vi "CT_OrganizeDischargeData.vi"(1 "Cap Discharge Array In":T1=[{"cap number and switch SN array"=[{"Switch SN"="SN_U", "Cap Number"=109.0}], "Rog"=enum."F240", "Delay"=enum."PreForm", "Power Supply"=enum."PS1"}, {"cap number and switch SN array"=[{"Switch SN"="SN_U", "Cap Number"=110.0}], "Rog"=enum."F180", "Delay"=enum."DB16", "Power Supply"=enum."PS2"}, {"cap number and switch SN array"=[{"Switch SN"="SN_U", "Cap Number"=111.0}], "Rog"=enum."F300", "Delay"=enum."DB16", "Power Supply"=enum."PS2"}, {"cap number and switch SN array"=[{"Switch SN"="SN_U", "Cap Number"=112.0}], "Rog"=enum."F000", "Delay"=enum."DB16", "Power Supply"=enum."PS2"}, {"cap number and switch SN array"=[{"Switch SN"="SN_U", "Cap Number"=113.0}], "Rog"=enum."F060", "Delay"=enum."DB16", "Power Supply"=enum."PS2"}, {"cap number and switch SN array"=[{"Switch SN"="SN_U", "Cap Number"=114.0}], "Rog"=enum."F120", "Delay"=enum."DB16", "Power Supply"=enum."PS2"}, {"cap number and switch SN array"=[{"Switch SN"="SN_U", "Cap Number"=115.0}], "Rog"=enum."F120", "Delay"=enum."DB16", "Power Supply"=enum."PS2"}, {"cap number and switch SN array"=[{"Switch SN"="SN_U", "Cap Number"=116.0}], "Rog"=enum."F060", "Delay"=enum."DB16", "Power Supply"=enum."PS2"}, {"cap number and switch SN array"=[{"Switch SN"="SN_U", "Cap Number"=117.0}], "Rog"=enum."F000", "Delay"=enum."DB16", "Power Supply"=enum."PS2"}, {"cap number and switch SN array"=[{"Switch SN"="SN_U", "Cap Number"=118.0}], "Rog"=enum."F300", "Delay"=enum."DB16", "Power Supply"=enum."PS2"}, {"cap number and switch SN array"=[{"Switch SN"="SN_U", "Cap Number"=119.0}], "Rog"=enum."F180", "Delay"=enum."DB16", "Power Supply"=enum."PS2"}, {"cap number and switch SN array"=[{"Switch SN"="SN_U", "Cap Number"=120.0}], "Rog"=enum."F240", "Delay"=enum."DB16", "Power Supply"=enum."PS2"}, {"cap number and switch SN array"=[{"Switch SN"="SN_U", "Cap Number"=121.0}], "Rog"=enum."F240", "Delay"=enum."DB16", "Power Supply"=enum."PS3"}, {"cap number and switch SN array"=[{"Switch SN"="SN_U", "Cap Number"=122.0}], "Rog"=enum."F300", "Delay"=enum."DB16", "Power Supply"=enum."PS3"}, {"cap number and switch SN array"=[{"Switch SN"="SN_U", "Cap Number"=123.0}], "Rog"=enum."F180", "Delay"=enum."DB16", "Power Supply"=enum."PS3"}, {"cap number and switch SN array"=[{"Switch SN"="SN_U", "Cap Number"=124.0}], "Rog"=enum."F240", "Delay"=enum."DB16", "Power Supply"=enum."PS3"}, {"cap number and switch SN array"=[{"Switch SN"="SN_U", "Cap Number"=125.0}], "Rog"=enum."DISC", "Delay"=enum."DB16", "Power Supply"=enum."PS3"}, {"cap number and switch SN array"=[{"Switch SN"="SN_U", "Cap Number"=126.0}], "Rog"=enum."F000", "Delay"=enum."DB16", "Power Supply"=enum."PS3"}, {"cap number and switch SN array"=[{"Switch SN"="SN_U", "Cap Number"=127.0}], "Rog"=enum."F060", "Delay"=enum."DB16", "Power Supply"=enum."PS3"}, {"cap number and switch SN array"=[{"Switch SN"="SN_U", "Cap Number"=128.0}], "Rog"=enum."DISC", "Delay"=enum."DB16", "Power Supply"=enum."PS3"}]) -> (0 "Discharge File Data":string[][](array[string]))   [LabVIEW 2016]
uses:
  CapDischargeCluster.ctl
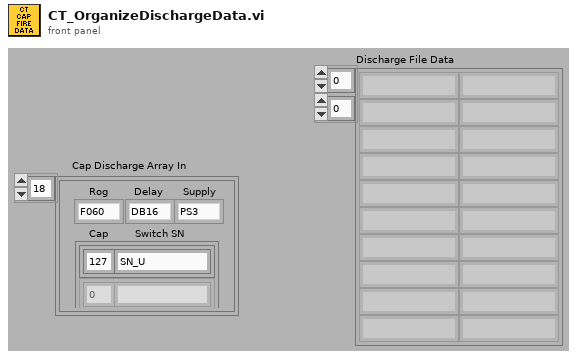
[diagram p1: front panel]
types:
  T1 = typedef "CapDischargeCluster.ctl" = cluster{"cap number and switch SN array":cluster{"Switch SN":string, "Cap Number":dbl}[], "Rog":enum16{"F000", "F060", "F120", "F180", "F240", "F300", "A015", "A045", "A075", "A105", "A135", "A165", "A195", "A225", "A255", "A285", "A315", "A345", "Snip", "DISC"}, "Delay":enum16{"DB00", "DB01", "DB02", "DB03", "DB04", "DB05", "DB06", "DB07", "DB08", "DB09", "DB10", "DB11", "DB12", "DB13", "DB14", "DB15", "DB16", "DB17", "DB18", "DB19", "DB20", "DB21", "DB22", "DB23", "DB24", "DB25", "DB26", "DB27", "DB28", "DB29", "DB30", "PreForm", "Form"}, "Power Supply":enum16{"PS1", "PS2", "PS3", "PS5", "PS6", "PS4"}}[]
  T2 = enum16{"F000", "F060", "F120", "F180", "F240", "F300", "A015", "A045", "A075", "A105", "A135", "A165", "A195", "A225", "A255", "A285", "A315", "A345", "Snip", "DISC"}
  T3 = enum16{"DB00", "DB01", "DB02", "DB03", "DB04", "DB05", "DB06", "DB07", "DB08", "DB09", "DB10", "DB11", "DB12", "DB13", "DB14", "DB15", "DB16", "DB17", "DB18", "DB19", "DB20", "DB21", "DB22", "DB23", "DB24", "DB25", "DB26", "DB27", "DB28", "DB29", "DB30", "PreForm", "Form"}
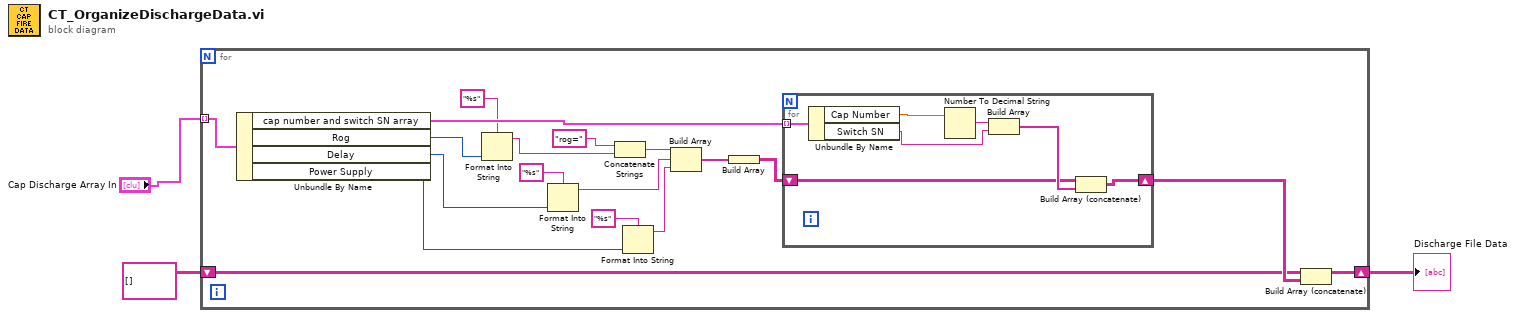
[diagram p0: block diagram]
diagram:
  n1 = for {
    tunnel: "Cap Discharge Array In" -> [w21] mode=indexing
    shift-right: [w18] -> w2
    shift-left: string[][] [] -> [w17]
    n2 = Unbundle By Name(w21) -> ("cap number and switch SN array"=w20:cluster{"Switch SN":string, "Cap Number":dbl}[], "Rog"=w16:T2, "Delay"=w13:T3, "Power Supply"=w5:enum16{"PS1", "PS2", "PS3", "PS5", "PS6", "PS4"})
    n3 = Format Into String(format string="%s", w16) -> (resulting string=w11:string)  [unwired: 2 in, 1 out]
    n4 = Format Into String(format string="%s", w13) -> (resulting string=w10:string)  [unwired: 2 in, 1 out]
    n5 = Concatenate Strings("rog=" ("string"), w11) -> (w9:string)
    n6 = Format Into String(format string="%s", w5) -> (resulting string=w4:string)  [unwired: 2 in, 1 out]
    n7 = Build Array(w9, w10, w4) -> (w8:string[])
    n8 = Build Array(w8) -> (w7:string[][])
    n9 = for {
      tunnel: w20 -> [w28] mode=indexing
      shift-right: [w23] -> w19
      shift-left: w7 -> [w22]
      n10 = Unbundle By Name(w28) -> ("Cap Number"=w26:dbl, "Switch SN"=w25:string)
      n11 = Number To Decimal String(number=w26) -> (decimal integer string=w27:string)  [unwired: 1 in]
      n12 = Build Array(w27, w25) -> (w24:string[])
      n13 = Build Array (concatenate)(w22, w24) -> (w23:string[][])
    }
    n14 = Build Array (concatenate)(w17, w19) -> (w18:string[][])
  }
  "Discharge File Data" <- w2
